vi "Check for Duplicate Stream IDs.vi"(8 "error in (no error)":errorcluster, 11 "stream-sorted transfers in":T1[](array[typedef])) -> (0 "error out":errorcluster, 3 "stream-sorted transfers out":T1[](array[typedef]))   [LabVIEW 2017, in "PXImc.lvlib" / "PXImc Transceiver.lvclass"]
uses:
  PXImc Transceiver.lvclass
  PXImc Transfer Data.ctl
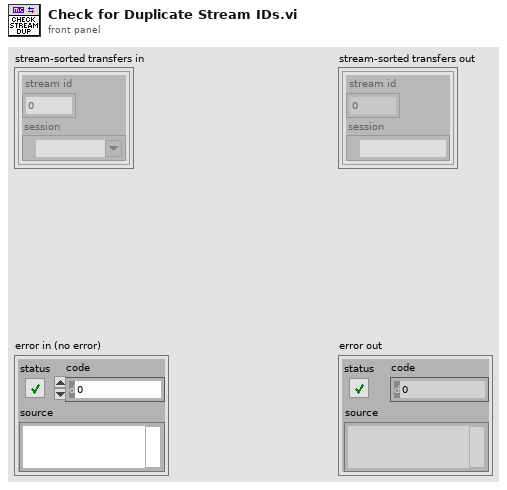
[diagram p1: front panel]
types:
  T1 = typedef "PXImc.lvlib/PXImc Transceiver.lvclass/PXImc Transfer Data.ctl" = cluster{"stream id":u16, "session":refnum<k21>}
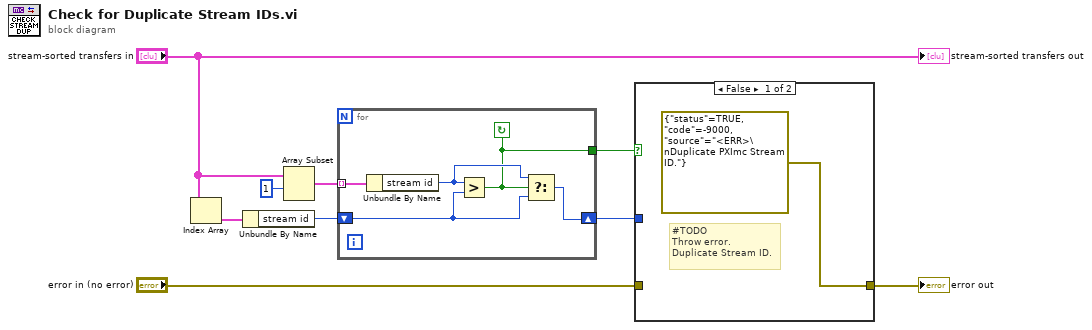
[diagram p0: block diagram]
diagram:
  n1 = Index Array(array="stream-sorted transfers in") -> (element=w9:T1)  [unwired: 1 in]
  n2 = Unbundle By Name(w9) -> ("stream id"=w8:u16)
  n3 = Array Subset(array="stream-sorted transfers in", index=1) -> (w6:T1[])  [unwired: 1 in]
  n4 = for {
    tunnel: w6 -> [w14] mode=indexing
    shift-right: [w11] -> w2
    shift-left: w8 -> [w12]
    tunnel: [w10] -> w5
    stop <- w10 continue-if-true
    n5 = Unbundle By Name(w14) -> ("stream id"=w13:u16)
    n6 = Greater?(x=w13, y=w12) -> (0:w10:bool)
    n7 = Select(t=w13, s=w10, f=w12) -> (s? t:f=w11:u16)
  }
  n8 = case shown="False" w5 {
    tunnel: "error in (no error)" -> [_ w16]
    tunnel: [errorcluster {"status"=TRUE, "code"=-9000, "source"="<ERR>\nDuplicate PXImc Stream ID."} ("error in (no error)") w16] -> w3
    tunnel: w2 -> [_ _]
    frame False {
      # "#TODO\nThrow error.\nDuplicate Stream ID."
    }
    frame True {
    }
  }
  "error out" <- w3
  "stream-sorted transfers out" <- "stream-sorted transfers in"
